vi "Configure Normal Current Range.vi"(8 "error in":errorcluster, 9 "Range":enum16{"AUTO", "HIGH", "LOW"}(ring), 10 "Phase":enum16{"A", "B", "C", "ALL"}(ring), 11 "VISA resource name":refnum<visa-resource-name>) -> (0 "error out":errorcluster, 3 "VISA resource name out":refnum<visa-resource-name>)   [LabVIEW 2020, in "IT-M7700.lvlib"]
doc: "This command is used to set the current range.\n<b>Phase</b>\n0: A\n1: B\n2: C\n3: ALL\n<b>Range</b>\n0: AUTO\n1: HIGH\n2: LOW"
uses:
  <instrlib>/IT-M7700/IT-M7700.lvlib
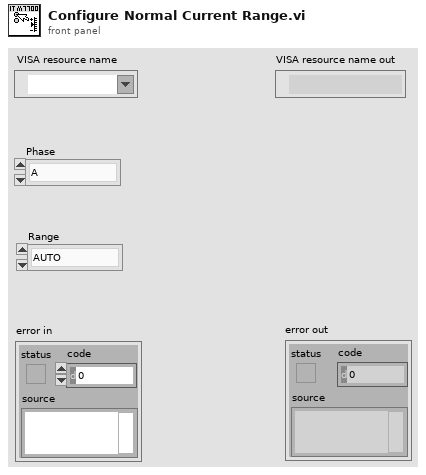
[diagram p1: front panel]
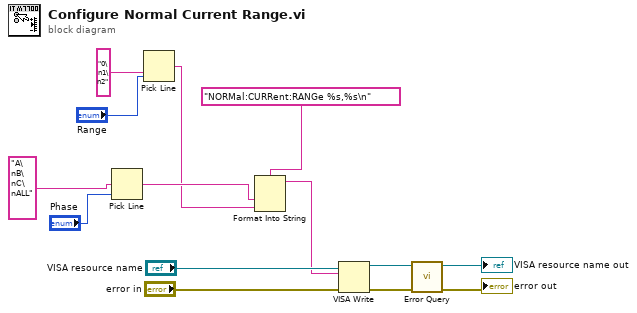
[diagram p0: block diagram]
diagram:
  n1 = Pick Line(multi-line string="A\nB\nC\nALL" ("多行字符串"), line index="Phase") -> (output string=w2:string)  [unwired: 1 in]
  n2 = Pick Line(multi-line string="0\n1\n2" ("多行字符串"), line index="Range") -> (output string=w1:string)  [unwired: 1 in]
  n3 = Format Into String(format string="NORMal:CURRent:RANGe %s,%s\n", w2, w1) -> (resulting string=w12:string)  [unwired: 2 in, 1 out]
  n4 = VISA Write(VISA resource name="VISA resource name", write buffer=w12, error in (no error)="error in") -> (VISA resource name out=w11:refnum<visa-resource-name>, error out=w10:errorcluster)  [unwired: 1 out]
  n5 = call <instrlib>:"Error Query.vi"("error in"=w10, "VISA resource name"=w11) -> ("error out"=→"error out":errorcluster, "VISA resource name out"=→"VISA resource name out":refnum<visa-resource-name>)  [unwired: 6 in, 2 out]
